vi "Close.vi"(8 "error in":errorcluster, 11 "Scope VISA CFG in":refnum<class "Scope VISA CFG.lvclass">) -> (0 "error out":errorcluster, 3 "Scope VISA CFG out":refnum<class "Scope VISA CFG.lvclass">)   [LabVIEW 2023, in "HAL.lvlib" / "Scope VISA.lvlib" / "Scope VISA CFG.lvclass"]
uses:
  Scope VISA CFG.lvclass
  Scope VISA CFG.lvclass/Scope VISA CFG.ctl
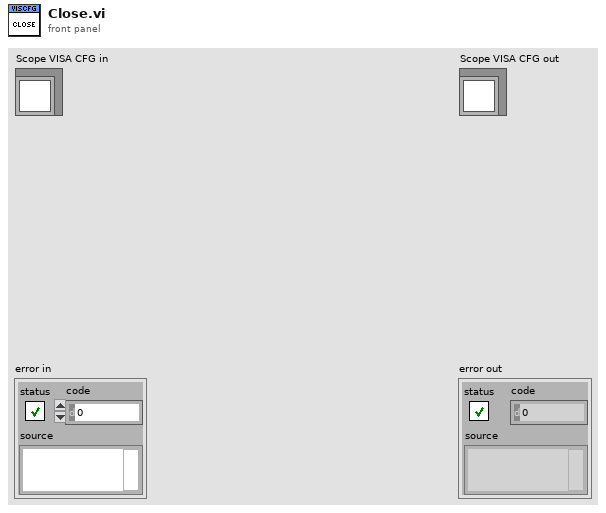
[diagram p1: front panel]
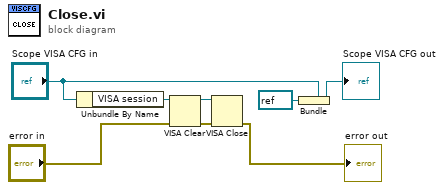
[diagram p0: block diagram]
diagram:
  n1 = Unbundle By Name("Scope VISA CFG in") -> ("VISA session"=w4:refnum<visa-resource-name>)
  n2 = VISA Clear(VISA resource name=w4, error in (no error)="error in") -> (VISA resource name out=w3:refnum<visa-resource-name>, error out=w5:errorcluster)
  n3 = VISA Close(VISA resource name=w3, error in (no error)=w5) -> (error out=→"error out":errorcluster)
  n4 = Bundle(cluster="Scope VISA CFG in", refnum<visa-resource-name> refnum ("VISA session")) -> (→"Scope VISA CFG out":refnum<class "Scope VISA CFG.lvclass">)
